vi "Enqueue.vi"(8 "error in (no error)":errorcluster, 9 "Message Priority (Normal)":T1=enum."Normal", 10 "Message":refnum<class "Message.lvclass">, 11 "Message Enqueuer in":refnum<class "Message Enqueuer.lvclass">) -> (0 "error out":errorcluster, 3 "Message Enqueuer out":refnum<class "Message Enqueuer.lvclass">)   [LabVIEW 2013, in "Actor Framework.lvlib" / "Message Enqueuer.lvclass"]
doc: "(<B>Filename</B>: Actor Framework.lvlib:Message Enqueuer.lvclass:Enqueue.vi)\n\nSends a message.\n\nIn most cases, instead of using this method, National Instruments recommends using the Actor Framework Message Maker dialog box. This dialog box helps you create the code that defines and sends the message. Use the Enqueue VI only if the VI that creates the message is not the one that sends it."
uses:
  <vilib>/ActorFramework/Message Enqueuer/Message Enqueuer.lvclass
  <vilib>/ActorFramework/Message/Message.lvclass
  <vilib>/ActorFramework/Message Enqueuer/Message Priority.ctl
  <vilib>/ActorFramework/Message Enqueuer/Message Enqueuer.lvclass/Message Enqueuer.ctl
  <vilib>/ActorFramework/Message Priority Queue/Message Priority Queue.lvclass
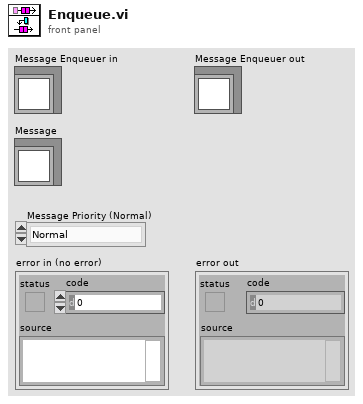
[diagram p1: front panel]
types:
  T1 = typedef "Actor Framework.lvlib/Message Enqueuer.lvclass/Message Priority.ctl" = enum16{"Low", "Normal", "High"}
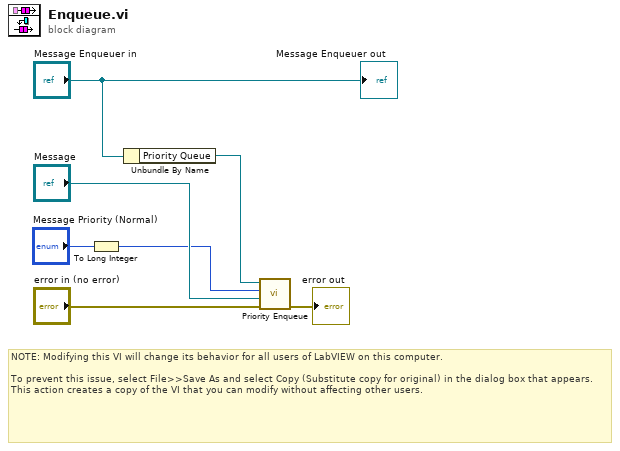
[diagram p0: block diagram]
diagram:
  # "NOTE: Modifying this VI will change its behavior for all users of LabVIEW on this computer.\n\nTo prevent this issue, select File>>Save As and select Copy (Substitute copy for original) in the dialog box that appears. This action creates a copy of the VI that you can modify without affecting other users."
  n1 = To Long Integer(number="Message Priority (Normal)") -> (32bit integer=w2:i32)
  n2 = Unbundle By Name("Message Enqueuer in") -> ("Priority Queue"=w6:refnum<class "Message Priority Queue.lvclass">)
  n3 = call <vilib>:"Priority Enqueue.vi"("error in (no error)"="error in (no error)", "Message"="Message", "priority"=w2, "Priority Queue in"=w6) -> ("error out"=→"error out":errorcluster)  [unwired: 6 in, 1 out]
  "Message Enqueuer out" <- "Message Enqueuer in"
